vi "XY Graph Add Plot(s) with Name(s).vi"   [LabVIEW 2021, in "XY Graph Add-Ons.lvlib"]
uses:
  XY Graph Add-Ons.lvlib
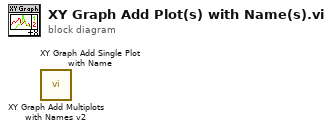
[diagram p0: block diagram]
diagram:
  n1 = call "XY Graph Add Multiplots with Names v2.vi"() -> ()  [unwired: 11 in, 5 out]
  n2 = call "XY Graph Add Single Plot with Name.vi"() -> ()  [unwired: 12 in, 4 out]
